vi "Module - Modbus Client.vi"() -> ()   [LabVIEW 2020]
uses:
  Control/State - Modbus Client.ctl
  <vilib>/NI/Modbus Library/API/Master/Modbus Master.lvclass
  Control/Data Struct - Display Data.ctl
  Control/Data Struct - SB.ctl
  Control/Data Struct - Bank.ctl
  Control/Data Struct - SI.ctl
  Control/Data Struct - PM.ctl
  Control/Device Name.ctl
  Control/State - eFGV.ctl
  Control/Config File Selection.ctl
  Control/Data Struct - Modbus Status.ctl
  Control/Data Struct - Modbus Reply.ctl
  <vilib>/NI/Modbus Library/API/Wrapper/Create TCP Master.vi
  <vilib>/NI/Modbus Library/API/Wrapper/API Main.lvlib
panel:
  out "error out":errorcluster
  in  "error in (no error)":errorcluster
types:
  T1 = typedef "Data Struct - Display Data.ctl" = cluster{"SB-01":T2, "SB-02":T2, "Bank-01":T3, "Bank-02":T3, "SI-M":T4, "SI-01":T4, "PM-01":T5}
  T2 = typedef "Data Struct - SB.ctl" = cluster{"Pac":dbl, "A.Vdc":dbl, "A.Idc":dbl, "B.Vdc":dbl, "B.Idc":dbl}
  T3 = typedef "Data Struct - Bank.ctl" = cluster{"SOC":dbl, "V_Bat":dbl, "I_Bat":dbl, "T_Bat":dbl}
  T4 = typedef "Data Struct - SI.ctl" = cluster{"Pac":dbl, "L1":dbl, "L2":dbl, "L3":dbl, "Freq":dbl}
  T5 = typedef "Data Struct - PM.ctl" = cluster{"Pac":dbl, "Vac":dbl, "Iac":dbl, "Freq":dbl}
  T6 = typedef "Device Name.ctl" = enum16{"SB-01", "SB-02", "BANK-01", "BANK-02", "SI-M", "SI-01", "PM-01"}
  T7 = cluster{"Timeout":i32, "Modbus Instance":refnum<class "Modbus Master.lvclass">, "Modbus Status":bool[], "Data Struct - All":T1, "Modbus Req":T6, "Modbus Setting":string[][], "register values":u16[][]}
  T8 = typedef "State - Modbus Client.ctl" = enum16{"Init module", "Register event", "Read Config File", "Idle", "Open Modbus Instance", "Read Modbus", "Process Register", "Send Reply", "Close Modbus Instance", "Unregister event", "Close module"}
  T9 = typedef "Config File Selection.ctl" = enum16{"Modbus", "SQL", "General"}
  T10 = typedef "Data Struct - Modbus Status.ctl" = cluster{"Modbus Req":T6, "Status":bool}
  T11 = typedef "State - eFGV.ctl" = enum16{"Init", "Read", "Write", "Close"}
  T12 = typedef "Data Struct - Modbus Reply.ctl" = cluster{"Modbus Req":T6, "Output Data":dbl[]}
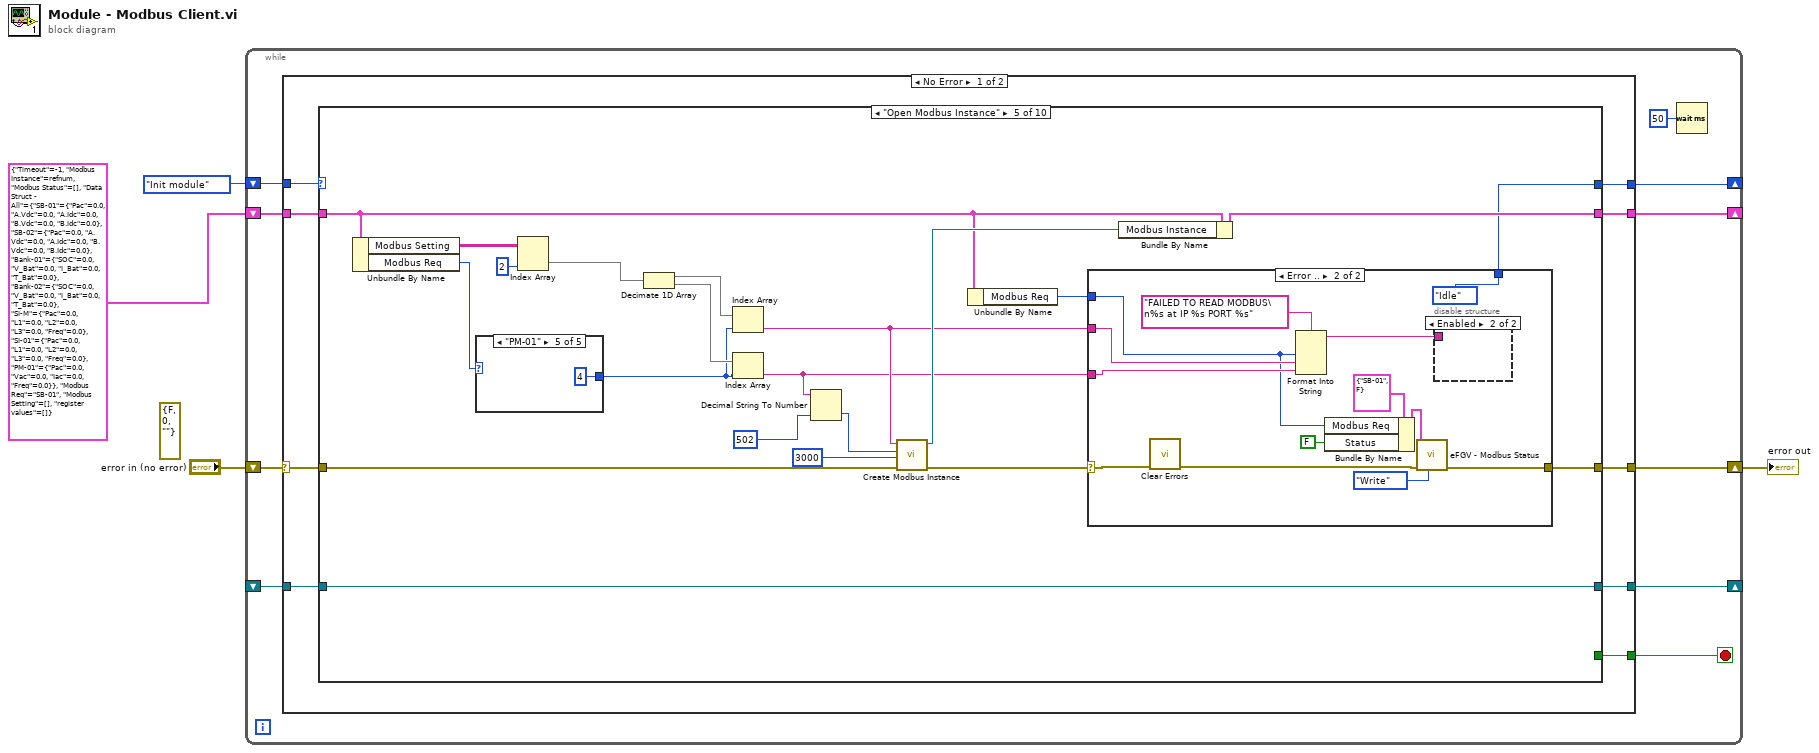
[diagram p0: block diagram]
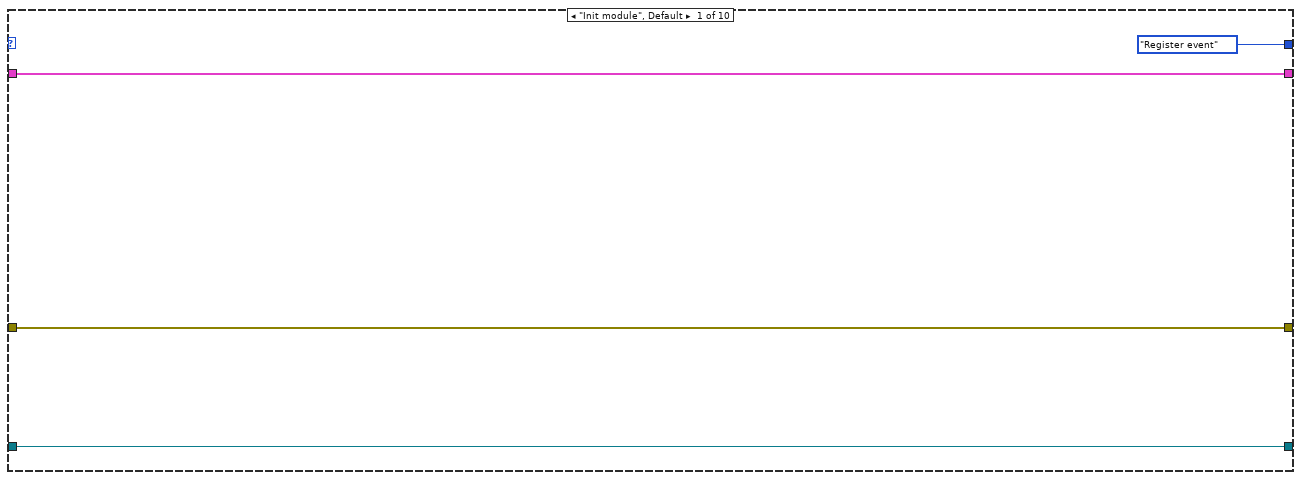
[diagram p2: hidden frame]
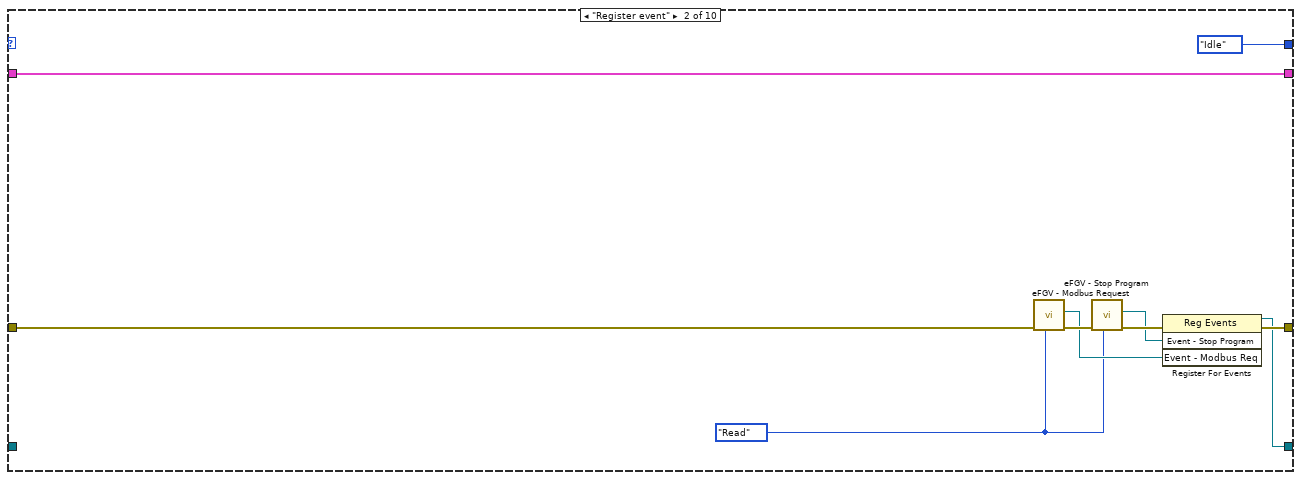
[diagram p3: hidden frame]
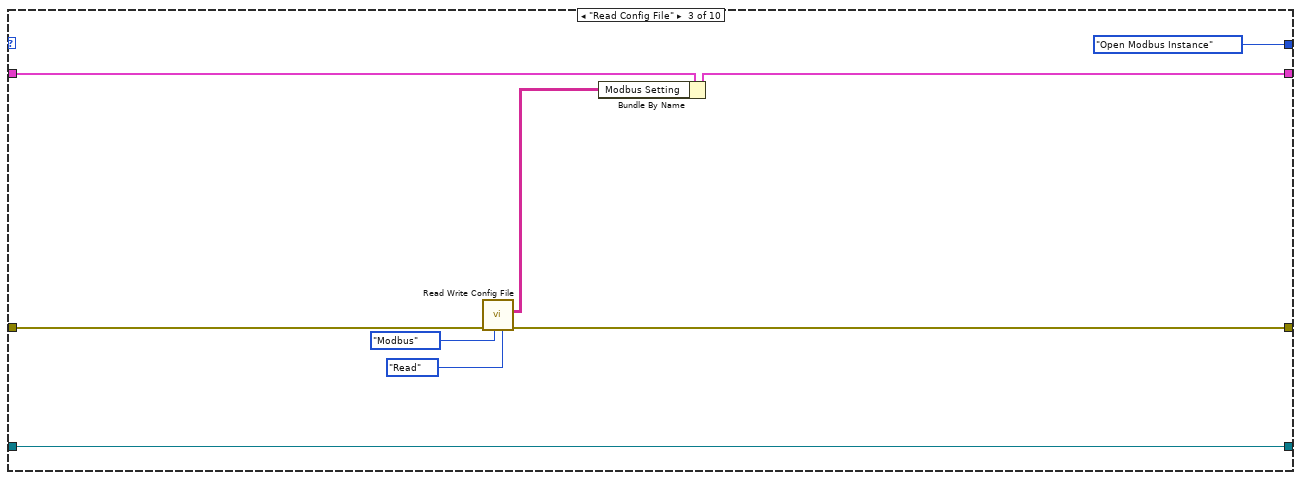
[diagram p4: hidden frame]
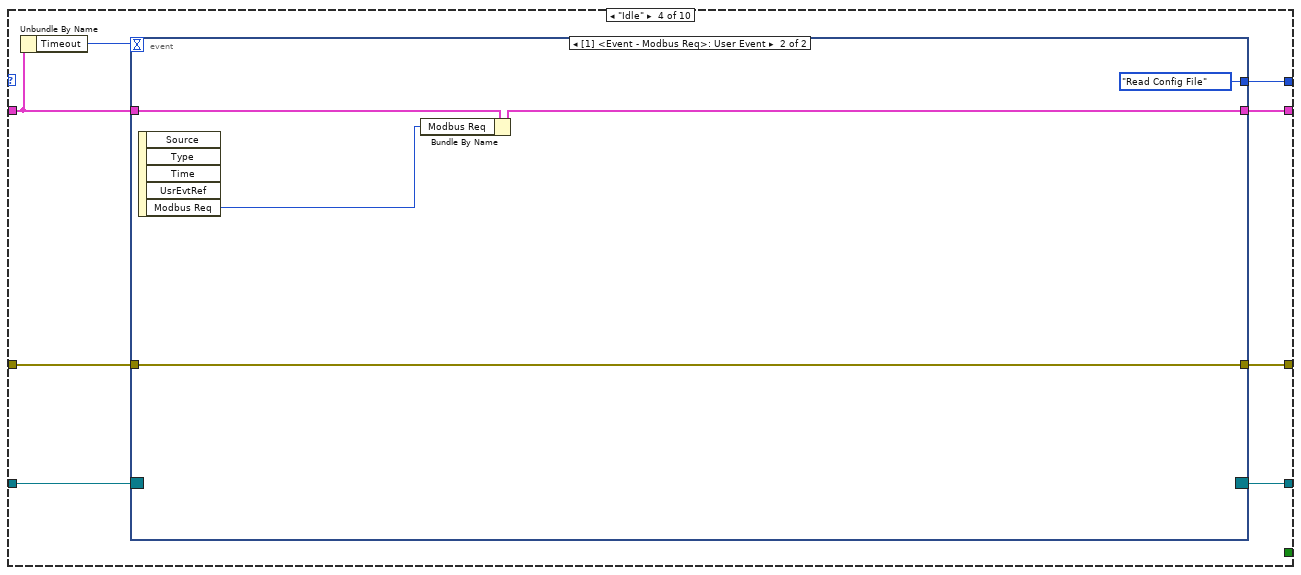
[diagram p5: hidden frame]
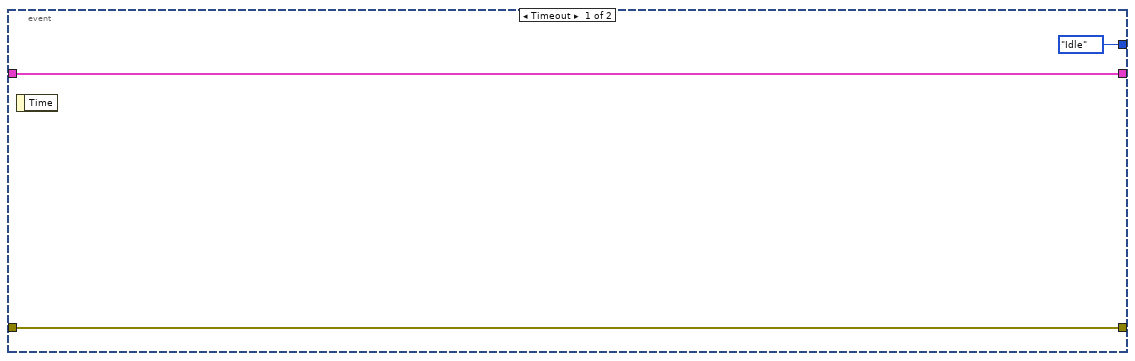
[diagram p6: hidden frame]
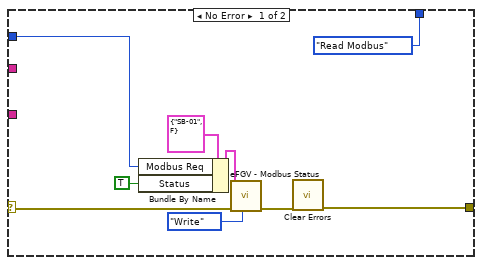
[diagram p7: hidden frame]
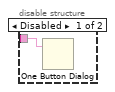
[diagram p8: hidden frame]
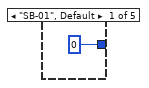
[diagram p9: hidden frame]
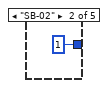
[diagram p10: hidden frame]
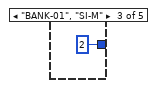
[diagram p11: hidden frame]
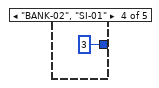
[diagram p12: hidden frame]
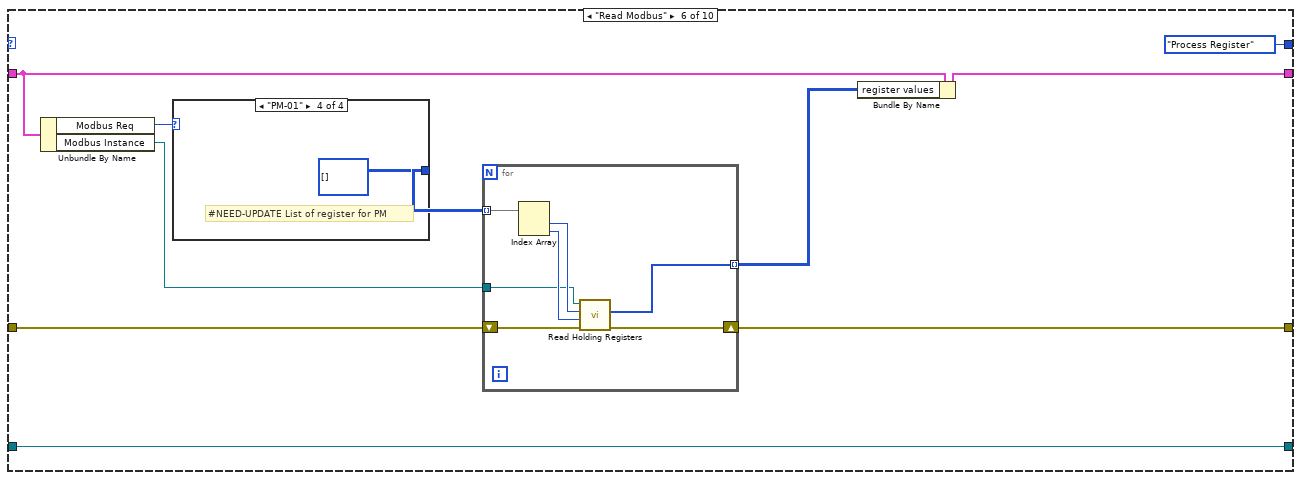
[diagram p13: hidden frame]
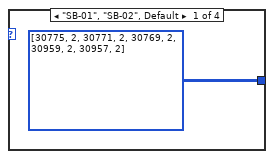
[diagram p14: hidden frame]
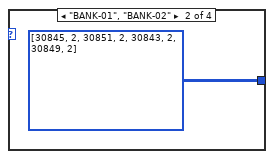
[diagram p15: hidden frame]
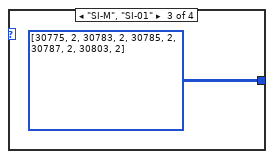
[diagram p16: hidden frame]
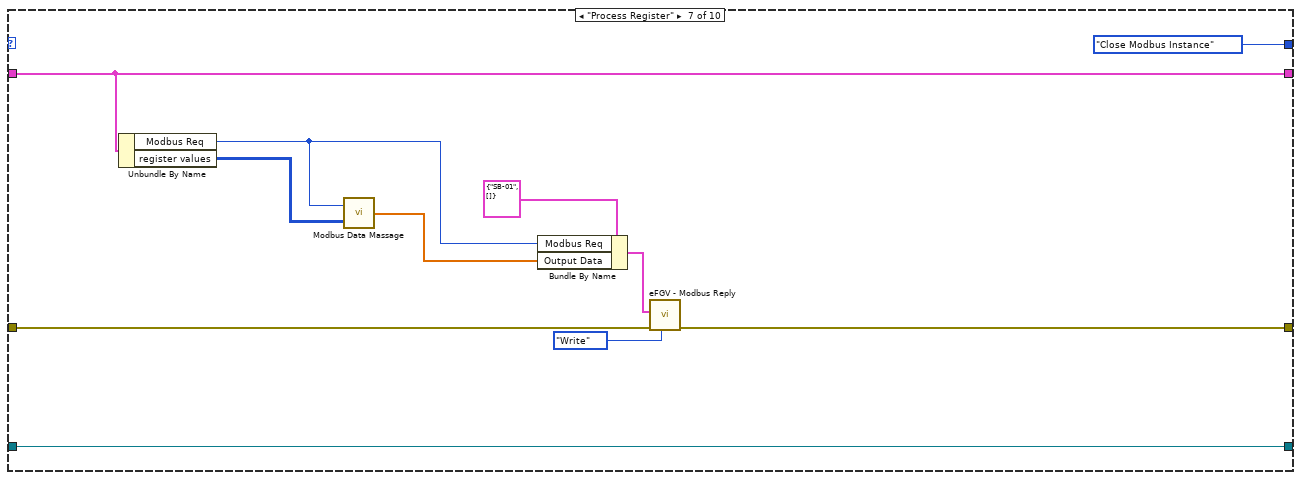
[diagram p17: hidden frame]
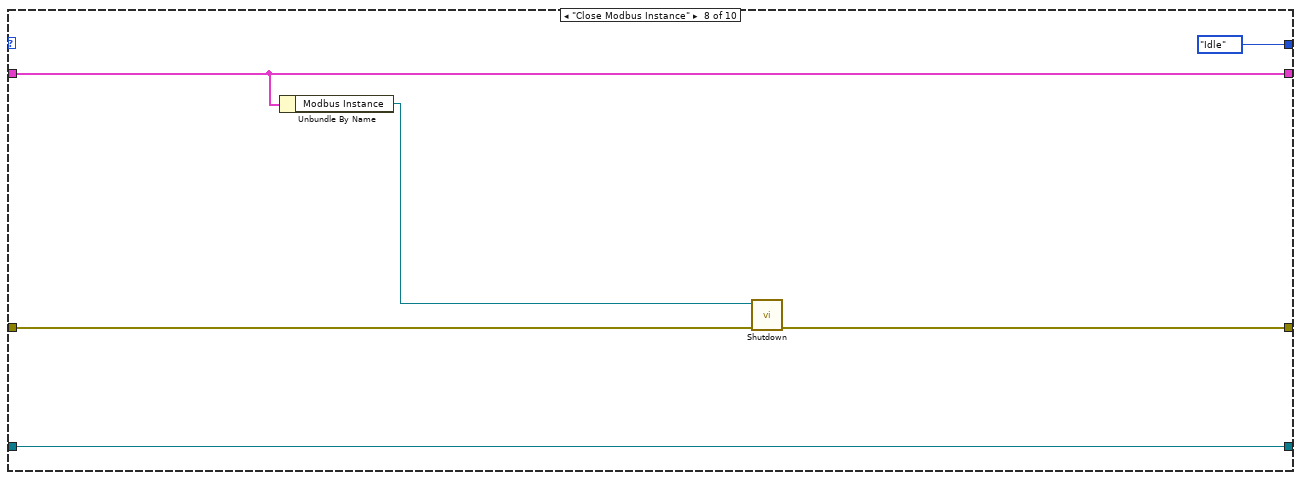
[diagram p18: hidden frame]
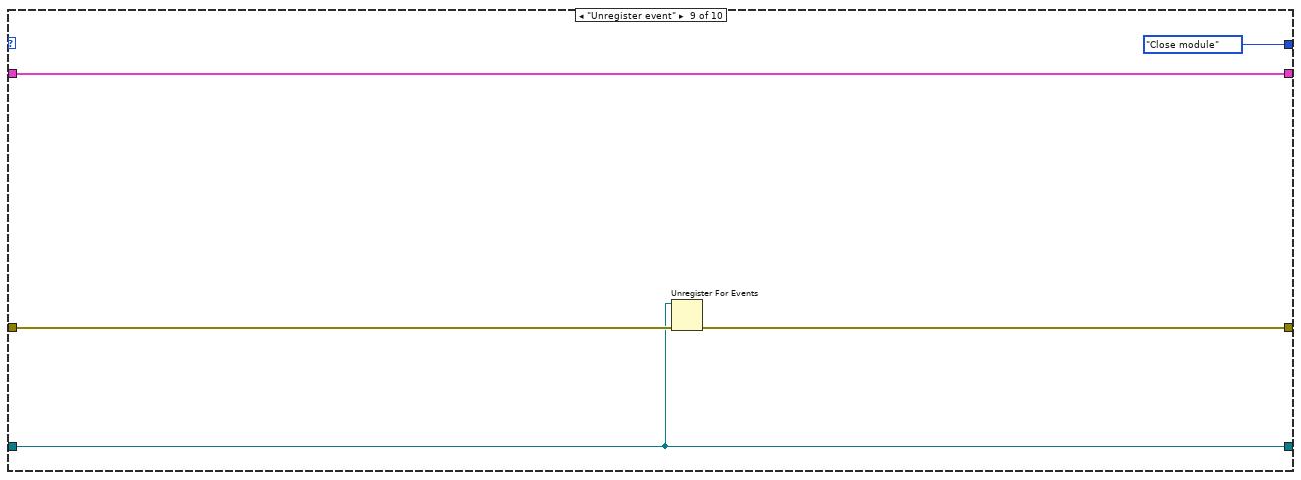
[diagram p19: hidden frame]
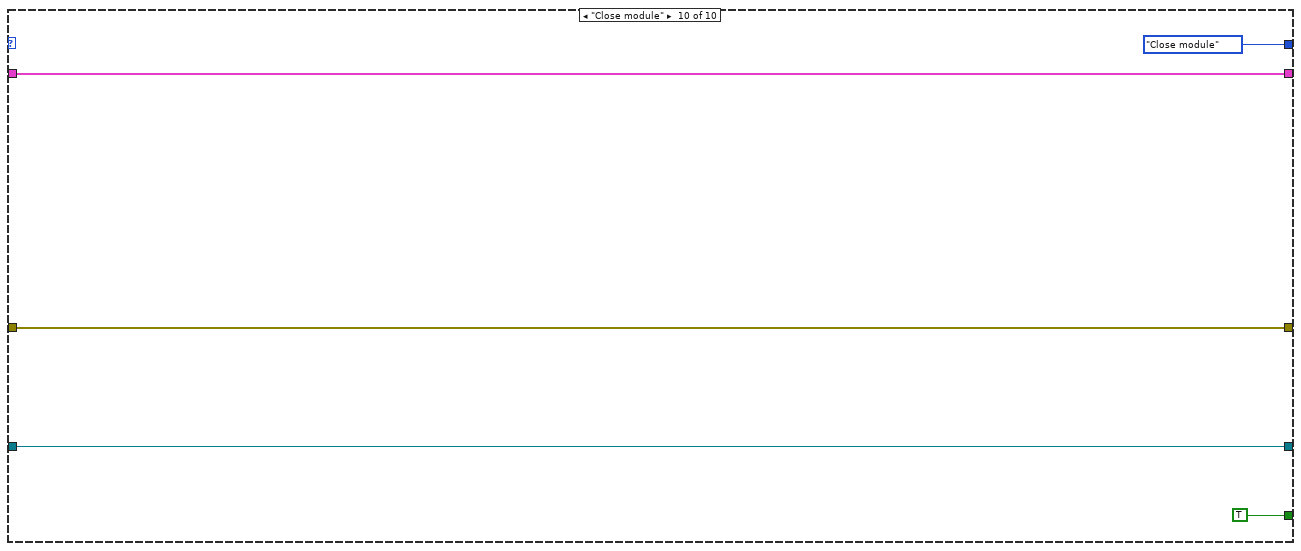
[diagram p20: hidden frame]
diagram:
  (unwired) errorcluster {"status"=FALSE, "code"=0, "source"=""} ("error in (no error)")
  n1 = while {
    shift-right: [w12] -> w3
    shift-left: "error in (no error)" -> [w14]
    shift-right: [w6] -> _
    shift-left: State_-_Modbus_Client."Init module" -> [w13]
    shift-right: [w11] -> _
    shift-left: _ -> [w10]
    shift-right: [w8] -> _
    shift-left: T7 {"Timeout"=-1, "Modbus Instance"=refnum, "Modbus Status"=[], "Data Struct - All"={"SB-01"={"Pac"=0.0, "A.Vdc"=0.0, "A.Idc"=0.0, "B.Vdc"=0.0, "B.Idc"=0.0}, "SB-02"={"Pac"=0.0, "A.Vdc"=0.0, "A.Idc"=0.0, "B.Vdc"=0.0, "B.Idc"=0.0}, "Bank-01"={"SOC"=0.0, "V_Bat"=0.0, "I_Bat"=0.0, "T_Bat"=0.0}, "Bank-02"={"SOC"=0.0, "V_Bat"=0.0, "I_Bat"=0.0, "T_Bat"=0.0}, "SI-M"={"Pac"=0.0, "L1"=0.0, "L2"=0.0, "L3"=0.0, "Freq"=0.0}, "SI-01"={"Pac"=0.0, "L1"=0.0, "L2"=0.0, "L3"=0.0, "Freq"=0.0}, "PM-01"={"Pac"=0.0, "Vac"=0.0, "Iac"=0.0, "Freq"=0.0}}, "Modbus Req"=enum."SB-01", "Modbus Setting"=[], "register values"=[]} -> [w9]
    stop <- w7 stop-if-true
    n2 = case shown="No Error" w14 {
      selector: w14 -> [w22 w164]
      tunnel: w13 -> [w23 _]
      tunnel: [w21 w163] -> w12
      tunnel: [w20 w162] -> w11
      tunnel: w10 -> [w19 w162]
      tunnel: w9 -> [w18 w161]
      tunnel: [w17 w161] -> w8
      tunnel: [w16 _] -> w7
      tunnel: [w15 State_-_Modbus_Client."Idle"] -> w6
      frame No Error {
        n3 = case shown="\"Open Modbus Instance\"" w23 {
          tunnel: w22 -> [w27 w28 w43 w51 w82 w117 w140 w146 w153 w159]
          tunnel: [w27 w37 w42 w48 w77 w112 w139 w144 w152 w159] -> w21
          tunnel: [w26 w36 w46 w49 w83 w121 w143 w149 w151 w158] -> w20
          tunnel: w19 -> [w26 _ w46 w50 w83 w121 w143 w149 w151 w158]
          tunnel: w18 -> [w25 w35 w45 w53 w68 w118 w142 w148 w154 w157]
          tunnel: [w25 w35 w39 w52 w79 w114 w142 w148 w154 w157] -> w17
          tunnel: [_ _ _ _ _ _ _ _ _ TRUE] -> w16
          tunnel: [State_-_Modbus_Client."Register event" State_-_Modbus_Client."Idle" State_-_Modbus_Client."Open Modbus Instance" w47 w69 State_-_Modbus_Client."Process Register" State_-_Modbus_Client."Close Modbus Instance" State_-_Modbus_Client."Idle" State_-_Modbus_Client."Close module" State_-_Modbus_Client."Close module"] -> w15
          frame "Init module", Default {
          }
          frame "Register event" {
            w29 = State_-_eFGV."Read" ("State - eFGV")
            n4 = call "eFGV - Modbus Request.vi"("State - eFGV"=w29, "error in (no error)"=w28) -> ("error out"=w32:errorcluster, "Event - Modbus Req"=w30:refnum<user-event>)  [unwired: 8 in]
            n5 = call "eFGV - Stop Program.vi"("State - eFGV"=w29, "error in (no error)"=w32) -> ("error out"=w33:errorcluster, "Event - Stop Program"=w31:refnum<user-event>)  [unwired: 8 in]
            n6 = register-events(error in=w33, w31, w30) -> (reference out=w36:refnum<event-registration>, error out=w37:errorcluster)  [unwired: 1 in]
          }
          frame "Read Config File" {
            n7 = call "Read Write Config File.vi"("Operation"=enum16{"Read", "Write"}."Read", "Config File"=Config_File_Selection."Modbus", "error in (no error)"=w43) -> ("error out"=w42:errorcluster, "Section-Key-Value Out"=w38:string[][])  [unwired: 7 in]
            n8 = Bundle By Name(cluster=w45, "Modbus Setting"=w38) -> (w39:T7)
          }
          frame "Idle" {
            n9 = Unbundle By Name(w53) -> ("Timeout"=w54:i32)
            n10 = event shown="[1] <Event - Modbus Req>: User Event" {
              selector: w50 -> [_ _]
              dyn-events: [_ _] -> w49
              timeout: w54 -> [_ _]
              tunnel: w53 -> [w57 w61]
              tunnel: [w57 w59] -> w52
              tunnel: w51 -> [w56 w60]
              tunnel: [w56 w60] -> w48
              tunnel: [State_-_Modbus_Client."Idle" State_-_Modbus_Client."Read Config File"] -> w47
              event Timeout {
                n11 = event-data() -> ()  [unwired: 1 in, 1 out]
              }
              event User Event {
                n12 = event-data() -> ("Modbus Req"=w58:T6)  [unwired: 1 in, 4 out]
                n13 = Bundle By Name(cluster=w61, "Modbus Req"=w58) -> (w59:T7)
              }
            }
          }
          frame "Open Modbus Instance" {
            n14 = Unbundle By Name(w68) -> ("Modbus Setting"=w81:string[][], "Modbus Req"=w73:T6)
            n15 = case shown="\"PM-01\"" w73 {
              tunnel: [0 ("index") 1 ("index") 2 ("index") 3 ("index") 4 ("index")] -> w71
              frame "SB-01", Default {
              }
              frame "SB-02" {
              }
              frame "BANK-01", "SI-M" {
              }
              frame "BANK-02", "SI-01" {
              }
              frame "PM-01" {
              }
            }
            n16 = Index Array(array=w81, index (col)=2 ("disabled index (col)")) -> (element=w76:string[])  [unwired: 1 in]
            n17 = Decimate 1D Array(w76) -> (w66:string[], w72:string[])
            n18 = Index Array(array=w66, index=w71) -> (element=w65:string)
            n19 = Index Array(array=w72, index=w71) -> (element=w64:string)
            n20 = Decimal String To Number(string=w64, default (0L)=u16 502 ("port (502)")) -> (number=w74:u16)  [unwired: 1 in, 1 out]
            n21 = call-poly <vilib>:"Create Modbus Instance.vi"("error in"=w82, "connect timeout ms"=3000, "port (502)"=w74, "address"=w65) -> ("error out"=w70:errorcluster, "TCP master instance"=w78:refnum<class "Modbus Master.lvclass">)  [unwired: 6 in]
            n22 = Unbundle By Name(w68) -> ("Modbus Req"=w67:T6)
            n23 = case shown="Error .." w70 {
              selector: w70 -> [w85 w94]
              tunnel: [w92 w95] -> w77
              tunnel: [State_-_Modbus_Client."Read Modbus" State_-_Modbus_Client."Idle"] -> w69
              tunnel: w67 -> [w84 w97]
              tunnel: w65 -> [_ w103]
              tunnel: w64 -> [_ w102]
              frame No Error {
                n24 = Bundle By Name(cluster=T10 {"Modbus Req"=enum."SB-01", "Status"=FALSE} ("Modbus Status"), "Modbus Req"=w84, "Status"=TRUE) -> (w88:T10)
                n25 = call "eFGV - Modbus Status.vi"("State - eFGV"=State_-_eFGV."Write", "error in (no error)"=w85, "Modbus Status"=w88) -> ("error out"=w86:errorcluster)  [unwired: 7 in, 1 out]
                n26 = call <vilib>:"Clear Errors.vi"("error in (no error)"=w86) -> ("error out"=w92:errorcluster)  [unwired: 5 in, 1 out]
              }
              frame Error {
                n27 = call <vilib>:"Clear Errors.vi"("error in (no error)"=w94) -> ("error out"=w93:errorcluster)  [unwired: 5 in, 1 out]
                n28 = Format Into String(format string="FAILED TO READ MODBUS\n%s at IP %s PORT %s", w97, w103, w102) -> (resulting string=w104:string)  [unwired: 2 in, 1 out]
                n29 = Bundle By Name(cluster=T10 {"Modbus Req"=enum."SB-01", "Status"=FALSE} ("Modbus Status"), "Modbus Req"=w97, "Status"=FALSE) -> (w98:T10)
                n30 = call "eFGV - Modbus Status.vi"("State - eFGV"=State_-_eFGV."Write", "error in (no error)"=w93, "Modbus Status"=w98) -> ("error out"=w95:errorcluster)  [unwired: 7 in, 1 out]
                n31 = disable-structure shown="Enabled" {
                  disable-tunnel: w104 -> [w106 _]
                  frame Disabled {
                    n32 = One Button Dialog(message=w106) -> ()  [unwired: 1 in, 1 out]
                  }
                  frame Enabled {
                  }
                }
              }
            }
            n33 = Bundle By Name(cluster=w68, "Modbus Instance"=w78) -> (w79:T7)
          }
          frame "Read Modbus" {
            n34 = Unbundle By Name(w118) -> ("Modbus Req"=w119:T6, "Modbus Instance"=w115:refnum<class "Modbus Master.lvclass">)
            n35 = case shown="\"PM-01\"" w119 {
              tunnel: [u16[][] [[30775, 2], [30771, 2], [30769, 2], [30959, 2], [30957, 2]] u16[][] [[30845, 2], [30851, 2], [30843, 2], [30849, 2]] u16[][] [[30775, 2], [30783, 2], [30785, 2], [30787, 2], [30803, 2]] u16[][] []] -> w116
              frame "SB-01", "SB-02", Default {
              }
              frame "BANK-01", "BANK-02" {
              }
              frame "SI-M", "SI-01" {
              }
              frame "PM-01" {
                # "#NEED-UPDATE List of register for PM"
              }
            }
            n36 = for {
              tunnel: w116 -> [w127] mode=indexing
              tunnel: [w124] -> w113 mode=indexing
              tunnel: w115 -> [w123]
              shift-right: [w122] -> w112
              shift-left: w117 -> [w128]
              n37 = Index Array(array=w127) -> (element #1=w126:u16, element #2=w125:u16)  [unwired: 2 in]
              n38 = call-dynamic "Read Holding Registers.vi"("error in"=w128, "number of inputs"=w125, "starting address"=w126, "Modbus master in"=w123) -> ("error out"=w122:errorcluster, "register values"=w124:u16[])  [unwired: 5 in, 1 out]
            }
            n39 = Bundle By Name(cluster=w118, "register values"=w113) -> (w114:T7)
          }
          frame "Process Register" {
            n40 = Unbundle By Name(w142) -> ("Modbus Req"=w135:T6, "register values"=w141:u16[][])
            n41 = call "Modbus Data Massage.vi"("register values"=w141, "Modbus Req"=w135) -> ("Output Data"=w134:dbl[])
            n42 = Bundle By Name(cluster=T12 {"Modbus Req"=enum."SB-01", "Output Data"=[]} ("Modbus Reply"), "Modbus Req"=w135, "Output Data"=w134) -> (w136:T12)
            n43 = call "eFGV - Modbus Reply.vi"("State - eFGV"=State_-_eFGV."Write", "error in (no error)"=w140, "Modbus Reply"=w136) -> ("error out"=w139:errorcluster)  [unwired: 7 in, 1 out]
          }
          frame "Close Modbus Instance" {
            n44 = Unbundle By Name(w148) -> ("Modbus Instance"=w145:refnum<class "Modbus Master.lvclass">)
            n45 = call-dynamic "Shutdown.vi"("error in"=w146, "Modbus master in"=w145) -> ("error out"=w144:errorcluster)  [unwired: 9 in]
          }
          frame "Unregister event" {
            n46 = Unregister For Events(event registration refnum=w151, error in=w153) -> (error out=w152:errorcluster)
          }
          frame "Close module" {
          }
        }
      }
      frame Error {
        n47 = call <vilib>:"Simple Error Handler.vi"("error in (no error)"=w164) -> ("error out"=w163:errorcluster)  [unwired: 4 in, 4 out]
      }
    }
    n48 = Wait (ms)(milliseconds to wait=u32 50) -> ()  [unwired: 1 out]
  }
  "error out" <- w3
